vi "Execute.vi"(4 "Position":i32, 6 "Assembly Type":string, 8 "Error In":errorcluster, 9 "Workspace":T1, 10 "Control In":T2={"I-O.lvclass"=refnum, "Gantry"=refnum, "Dispenser"="COM1"}, 11 "Dispense in":refnum<class "Dispense.lvclass">) -> (0 "Error Out":errorcluster, 2 "Control Out":T2={"I-O.lvclass"=refnum, "Gantry"=refnum, "Dispenser"="COM1"}, 3 "Dispense out":refnum<class "Dispense.lvclass">)   [LabVIEW 2021, in "Dispense.lvclass"]
uses:
  Dispense.lvclass
  Controller/Controllers.ctl
  Controller/I-O/I-O.lvclass
  C:/Program Files (x86)/Aerotech/A3200/LabVIEW/2010/Bin/Aerotech.A3200.dll
  Program Files (x86)/Aerotech/A3200/LabVIEW/2010/Bin/Aerotech.A3200.dll
  Workspace/Workspace.ctl
  Dispense.lvclass/Dispense.ctl
  Controller/Controller.lvclass
  Workspace/Fixture.lvclass
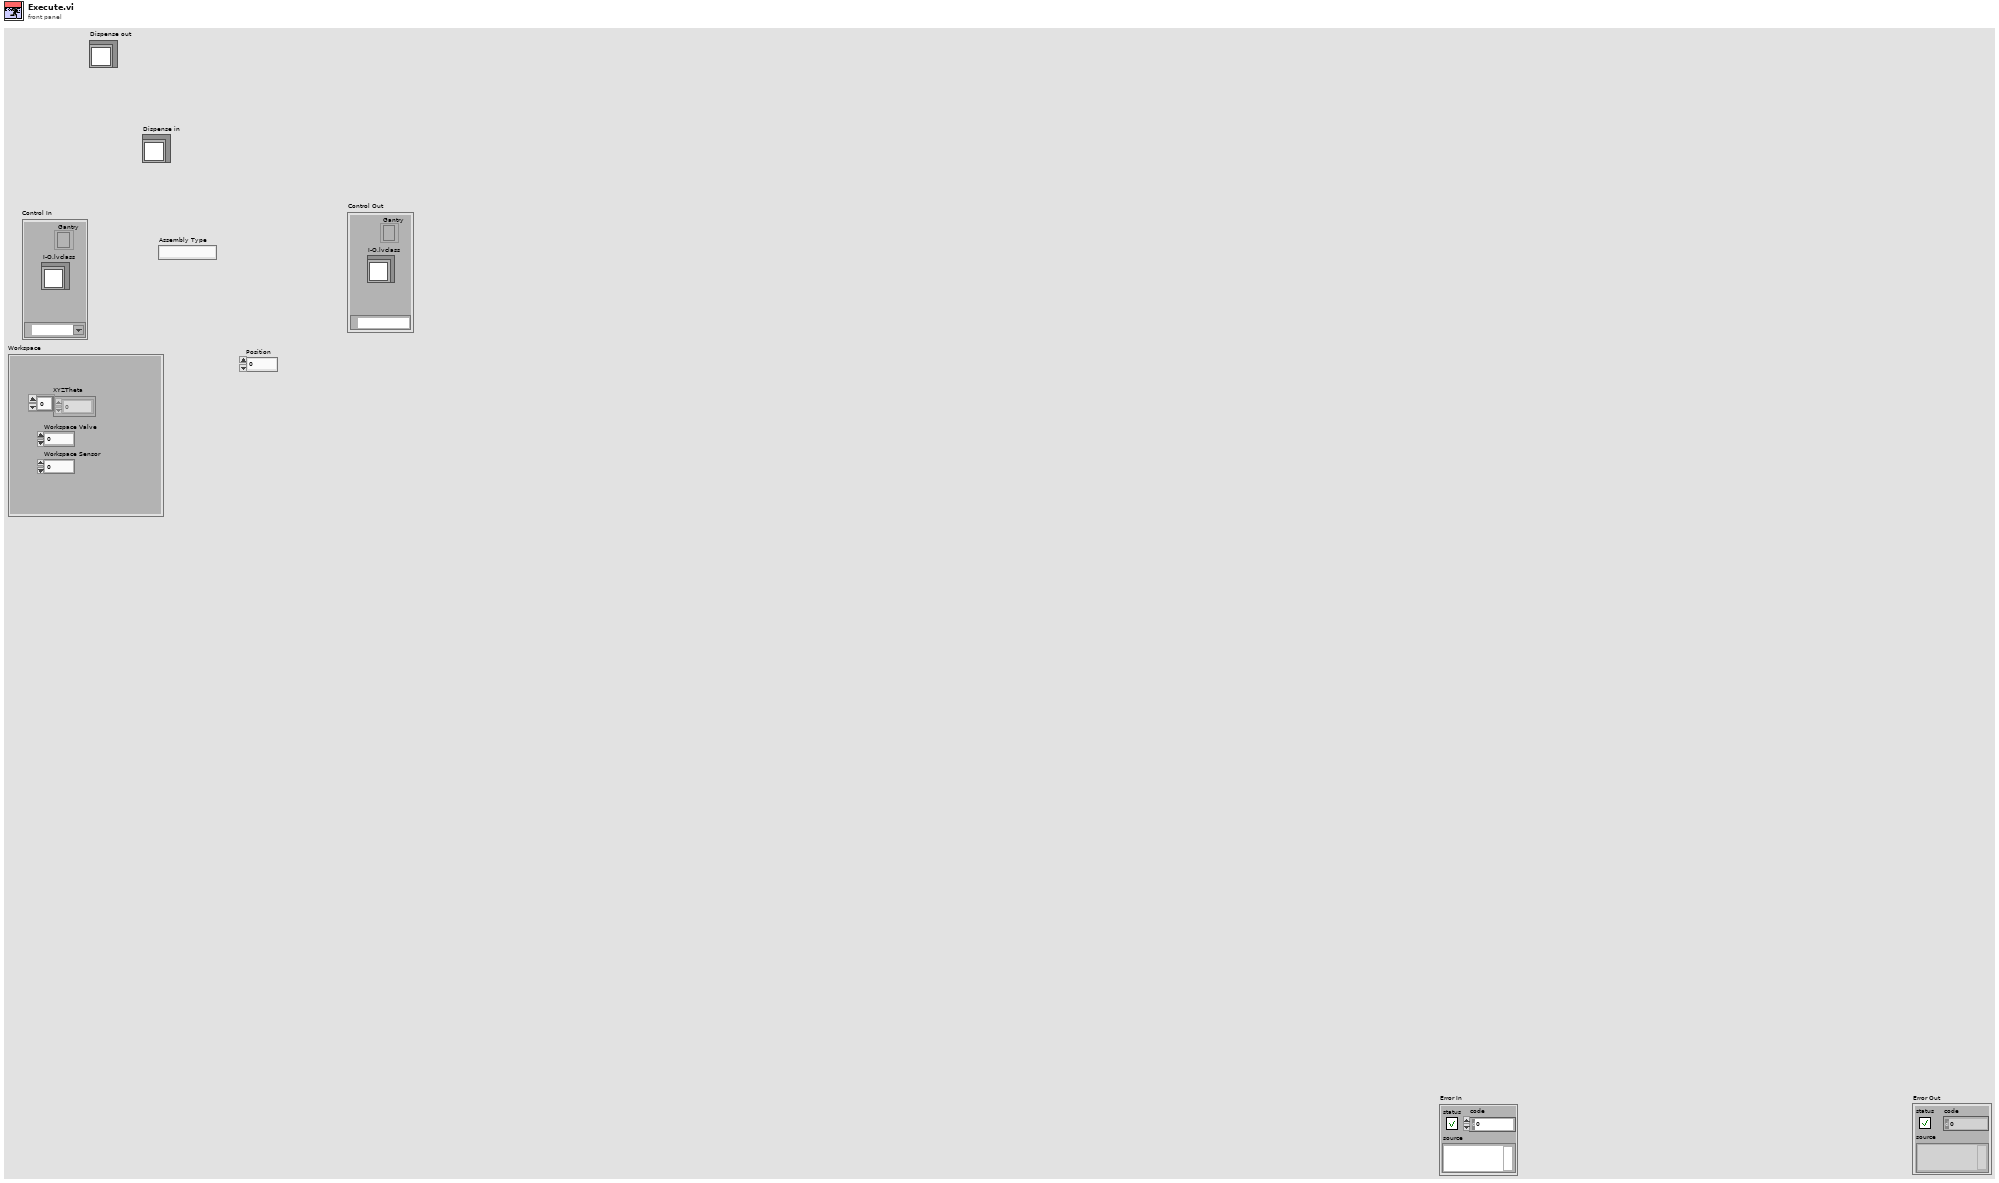
[diagram p1: front panel]
types:
  T1 = typedef "Fixture.lvclass/Workspace.ctl" = cluster{"XYZTheta":dbl[], "Workspace Valve":i32, "Workspace Sensor":i32}
  T2 = typedef "Controller.lvclass/Controllers.ctl" = cluster{"I-O.lvclass":refnum<class "I-O.lvclass">, "Gantry":refnum<k24>, "Dispenser":refnum<visa-resource-name>}
  T3 = cluster{"Time to Go Down":i32, "Time to Dispense":i32}[]
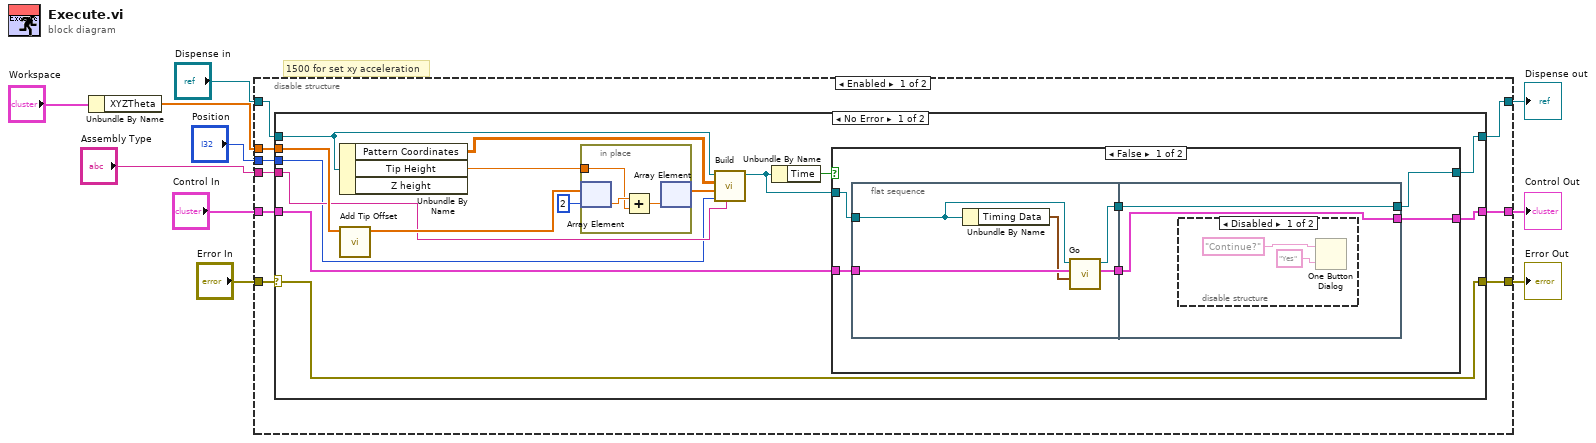
[diagram p0: block diagram]
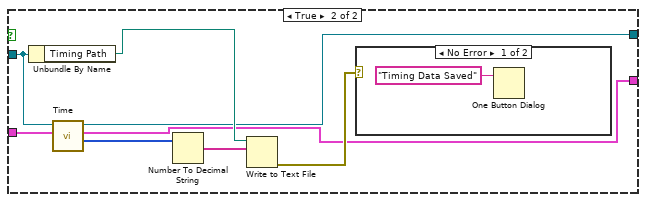
[diagram p3: hidden frame]
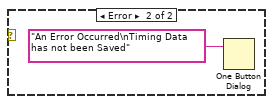
[diagram p4: hidden frame]
diagram:
  # "1500 for set xy acceleration"
  n1 = Unbundle By Name("Workspace") -> ("XYZTheta"=w4:dbl[])
  n2 = disable-structure shown="Enabled" {
    disable-tunnel: "Control In" -> [w19 w66]
    disable-tunnel: [w18 w66] -> w9
    disable-tunnel: "Dispense in" -> [w17 w68]
    disable-tunnel: "Error In" -> [w16 w67]
    disable-tunnel: [w15 w67] -> w6
    disable-tunnel: w4 -> [w14 _]
    disable-tunnel: [w13 w68] -> w3
    disable-tunnel: "Assembly Type" -> [w12 _]
    disable-tunnel: "Position" -> [w11 _]
    frame Enabled {
      n3 = case shown="No Error" w16 {
        selector: w16 -> [w34 w64]
        tunnel: w19 -> [w24 w65]
        tunnel: [w23 w65] -> w18
        tunnel: w17 -> [w27 w63]
        tunnel: [w34 w64] -> w15
        tunnel: w14 -> [w22 _]
        tunnel: [w32 w63] -> w13
        tunnel: w12 -> [w21 _]
        tunnel: w11 -> [w20 _]
        frame No Error {
          n4 = Unbundle By Name(w27) -> ("Pattern Coordinates"=w31:dbl[][], "Tip Height"=w28:dbl)  [unwired: 1 out]
          n5 = call "Add Tip Offset.vi"("XYZTheta"=w22) -> ("XYZTheta"=w26:dbl[])  [unwired: 10 in]
          n6 = in-place {
            in-place-border: w28 -> [w60]
            n7 = in-place-array #1(w26, 2) -> (w62:dbl)
            n8 = Add(x=w62, y=w60) -> (x+y=w61:dbl)
            n9 = in-place-array #1(w61) -> (w29:dbl[])  [unwired: 1 out]
          }
          n10 = call-dynamic "Build.vi"("Assembly Type"=w21, "Position"=w20, "XYZTheta"=w29, "Pattern Coordinates"=w31, "Dispense in"=w27) -> ("Dispense out"=w33:refnum<class "Dispense.lvclass">)  [unwired: 6 in]
          n11 = Unbundle By Name(w33) -> ("Time"=w25:bool)
          n12 = case shown="False" w25 {
            tunnel: w33 -> [w40 w51]
            tunnel: w24 -> [w39 w53]
            tunnel: [w37 w52] -> w23
            tunnel: [w38 w50] -> w32
            frame False {
              n13 = flat-sequence {
                tunnel: w40 -> [w45]
                tunnel: w39 -> [w44]
                tunnel: [w42] -> w36
                tunnel: [w41] -> w35
                tunnel: [w46] -> w37
                tunnel: [w47] -> w38
                tunnel: w36 -> [w47]
                tunnel: w35 -> [w46]
                frame #0 {
                  n14 = Unbundle By Name(w45) -> ("Timing Data"=w43:T3)
                  n15 = call-dynamic "Go.vi"("Timing Data"=w43, "Control In"=w44, "Dispense in"=w45) -> ("Control Out"=w41:T2, "Dispense Out"=w42:refnum<class "Dispense.lvclass">)  [unwired: 7 in]
                }
                frame #1 {
                  n16 = disable-structure shown="Disabled" {
                    frame Disabled {
                      n17 = One Button Dialog(message="Continue?", button name ("OK")="Yes") -> ()  [unwired: 1 out]
                    }
                    frame Enabled {
                    }
                  }
                }
              }
            }
            frame True {
              n18 = Unbundle By Name(w51) -> ("Timing Path"=w55:path)
              n19 = call-dynamic "Time.vi"("Control In"=w53, "Dispense in"=w51) -> ("Timing Data"=w54:i32[], "Control Out"=w52:T2, "Dispense out"=w50:refnum<class "Dispense.lvclass">)  [unwired: 6 in, 1 out]
              n20 = Number To Decimal String(number=w54) -> (decimal integer string=w56:string[])  [unwired: 1 in]
              n21 = Write to Text File(file (use dialog)=w55, text=w56) -> (error out=w57:errorcluster)  [unwired: 2 in, 2 out]
              n22 = case shown="No Error" w57 {
                frame No Error {
                  n23 = One Button Dialog(message="Timing Data Saved") -> ()  [unwired: 1 in, 1 out]
                }
                frame Error {
                  n24 = One Button Dialog(message="An Error Occurred\nTiming Data has not been Saved") -> ()  [unwired: 1 in, 1 out]
                }
              }
            }
          }
        }
        frame Error {
        }
      }
    }
    frame Disabled {
    }
  }
  "Control Out" <- w9
  "Error Out" <- w6
  "Dispense out" <- w3
